vi "預防保養設定次數To PLC.vi"(7 "Input Registers":u16[](array[numeric])=[0, 0, 0, 0, 0, 0, 0, 0], 8 "error in (no error)":errorcluster, 9 "Set Value Or Only Read":bool, 10 "Out starting address":u16=308, 11 "Set Item":string="$S2 Dect No") -> (0 "error out":errorcluster, 1 "Receive PLC Data":i32, 2 "data":i32)   [LabVIEW 2019]
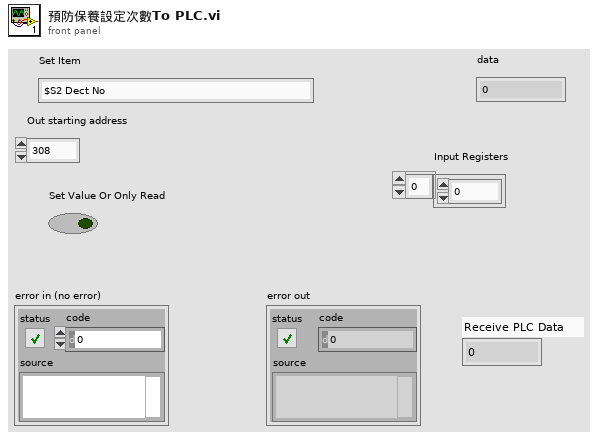
[diagram p1: front panel]
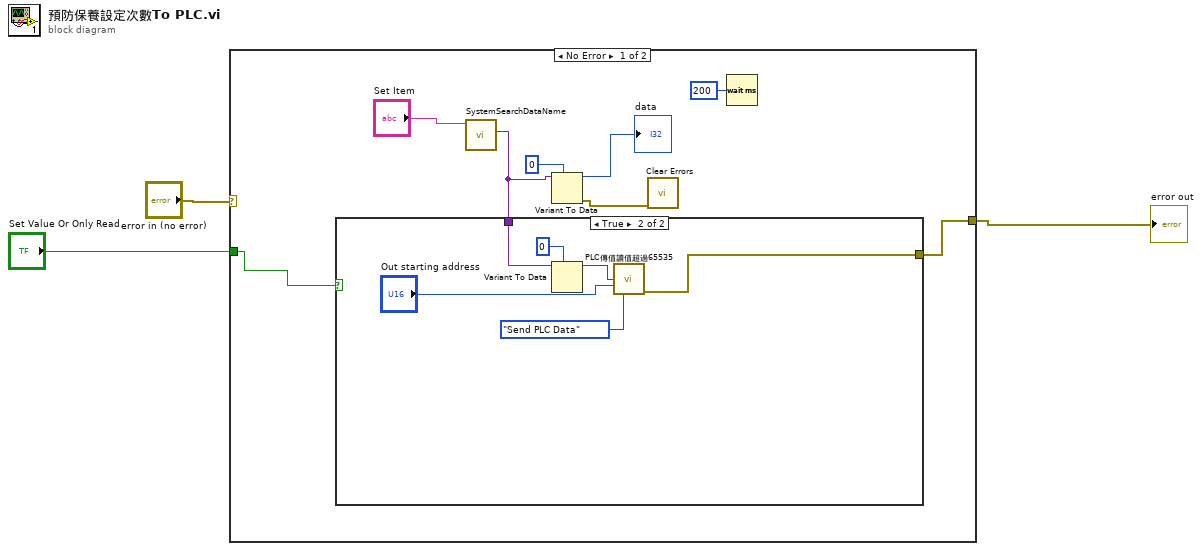
[diagram p0: block diagram]
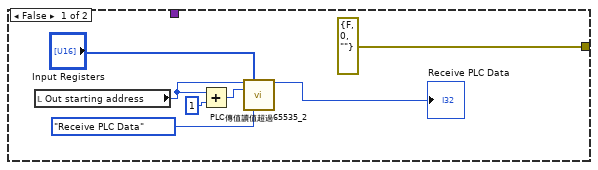
[diagram p2: hidden frame]
diagram:
  n1 = case shown="No Error" "error in (no error)" {
    selector: "error in (no error)" -> [_ w25]
    tunnel: [w10 w25] -> w2
    tunnel: "Set Value Or Only Read" -> [w9 _]
    frame No Error {
      n2 = call "SystemSearchDataName.vi"("element"="Set Item") -> ("variant"=w7:variant)  [unwired: 8 in, 2 out]
      n3 = case shown="True" w9 {
        tunnel: w7 -> [_ w24]
        tunnel: [errorcluster {"status"=FALSE, "code"=0, "source"=""} ("error out") w19] -> w10
        frame False {
          n4 = local read "Out starting address"() -> (w14:u16)
          n5 = Add(x=w14, y=u16 1) -> (x+y=w12:u16)
          n6 = call "PLC傳值讀值超過65535_2.vi"("Read PLC Reg Index0"=w14, "Input Registers"="Input Registers", "Read PLC Reg Index1"=w12, "Enum"=enum16{"Send PLC Data", "Receive PLC Data"}."Receive PLC Data") -> ("Receive PLC Data"=→"Receive PLC Data":i32)  [unwired: 9 in, 2 out]
        }
        frame True {
          n7 = Variant To Data(type=0 ("Numeric"), Variant=w24) -> (data=w21:i32)  [unwired: 1 in, 1 out]
          n8 = call "PLC傳值讀值超過65535.vi"("Out輸入值"=w21, "Out starting address"="Out starting address", "Enum"=enum16{"Send PLC Data", "Receive PLC Data"}."Send PLC Data") -> ("error out"=w19:errorcluster)  [unwired: 10 in, 2 out]
        }
      }
      n9 = Variant To Data(type=0 ("Numeric"), Variant=w7) -> (data=→"data":i32, error out=w5:errorcluster)  [unwired: 1 in]
      n10 = call <vilib>:"Clear Errors.vi"("error in (no error)"=w5) -> ()  [unwired: 5 in, 2 out]
      n11 = Wait (ms)(milliseconds to wait=u32 200) -> ()  [unwired: 1 out]
    }
    frame Error {
    }
  }
  "error out" <- w2
